vi "Arm_Control.vi"() -> ()   [LabVIEW 2012]
uses:
  StateMachineType.ctl
  Robot Global Data.vi
panel:
  in  "ArmBackSpeed":dbl=-0.32
  in  "ArmForwardSpeed":dbl=0.32
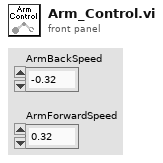
[diagram p1: front panel]
types:
  T1 = typedef "StateMachineType.ctl" = enum16{"Init", "Idle", "Start", "Do", "Stop"}
  T2 = typedef "WPI_MotorControlDeviceRef.ctl" = cluster{"DeviceStatus":errorcluster, "Type":enum16{"PWM", "CAN"}, "PWM":cluster{"Digital Module":T3, "PWM Channel":T4, "DeadBand":T5}, "CAN":cluster{"Device Number":u8, "Control Mode":T6, "Semaphore":T7, "Max Vout":dbl}, "Invert":bool, "TransformRef":T8, "InvTransformRef":T8}
  T3 = typedef "FPGA_TypedefDigitalModule.ctl" = enum16{"Digital Module 1", "Digital Module 2"}
  T4 = typedef "FPGA_DIOPWMChannel.ctl" = enum8{"PWM 1", "PWM 2", "PWM 3", "PWM 4", "PWM 5", "PWM 6", "PWM 7", "PWM 8", "PWM 9", "PWM 10", "Invalid"}
  T5 = typedef "WPI_PWMDeadband.ctl" = cluster{"Name":string, "maxPositivePwm":i32, "minPositivePwm":i32, "centerPwm":i32, "maxNegativePwm":i32, "minNegativePwm":i32, "angularRange":u16}
  T6 = typedef "WPI_CANJaguar_ControlMode.ctl" = enum8{"Percent VBus", "Current", "Speed", "Position", "Voltage"}
  T7 = typedef "Semaphore RefNum" = refnum<k1>
  T8 = typedef "WPI_PWMTransform_ConPane.ctl" = refnum<vi>
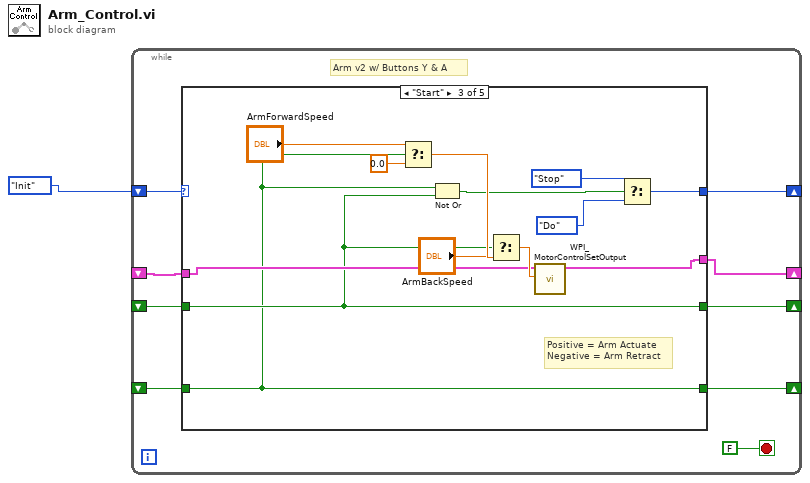
[diagram p0: block diagram]
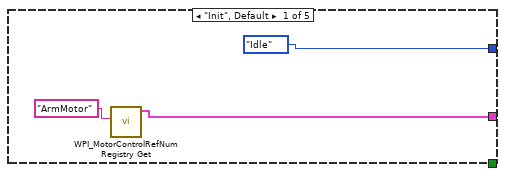
[diagram p2: hidden frame]
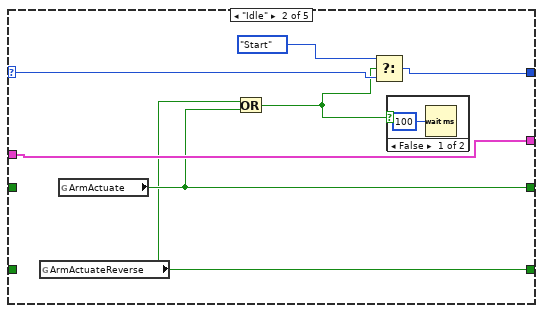
[diagram p3: hidden frame]
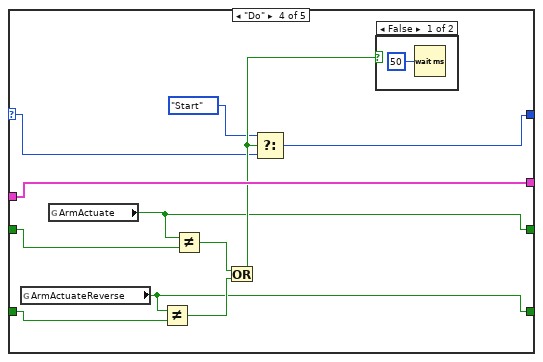
[diagram p5: hidden frame]
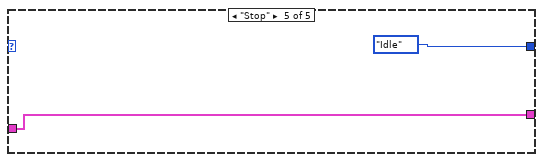
[diagram p7: hidden frame]
diagram:
  n1 = while {
    shift-right: [w6] -> _
    shift-left: _ -> [w9]
    shift-right: [w7] -> _
    shift-left: StateMachineType."Init" -> [w8]
    shift-right: [w4] -> _
    shift-left: _ -> [w2]
    shift-right: [w5] -> _
    shift-left: _ -> [w3]
    stop <- FALSE stop-if-true
    # "Arm v2 w/ Buttons Y & A"
    n2 = case shown="\"Start\"" w8 {
      selector: w8 -> [_ w20 _ w35 _]
      tunnel: w9 -> [_ w17 w24 w45 w47]
      tunnel: [StateMachineType."Idle" ("Enum") w18 w26 w39 StateMachineType."Idle" ("Enum")] -> w7
      tunnel: [w11 w17 w25 w45 w47] -> w6
      tunnel: [_ w15 w23 w38 _] -> w5
      tunnel: [_ w14 w22 w37 _] -> w4
      tunnel: w3 -> [_ _ w23 w44 _]
      tunnel: w2 -> [_ _ w22 w43 _]
      frame "Init", Default {
        n3 = call <vilib>:"WPI_MotorControlRefNum Registry Get.vi"("refnum name"="ArmMotor") -> ("MotorControlDevRef"=w11:T2)  [unwired: 9 in, 1 out]
      }
      frame "Idle" {
        n4 = global read "Robot Global Data.vi" "ArmActuateReverse"() -> (w14:bool)
        n5 = global read "Robot Global Data.vi" "ArmActuate"() -> (w15:bool)
        n6 = Or(x=w14, y=w15) -> (x .or. y?=w16:bool)
        n7 = Select(t=StateMachineType."Start" ("Enum"), s=w16, f=w20) -> (s? t:f=w18:T1)
        n8 = case shown="False" w16 {
          frame False {
            n9 = Wait (ms)(milliseconds to wait=u32 100) -> ()  [unwired: 1 out]
          }
          frame True {
          }
        }
      }
      frame "Start" {
        # "Positive = Arm Actuate\nNegative = Arm Retract"
        n10 = Select(t="ArmForwardSpeed", s=w22, f=0.0) -> (s? t:f=w34:dbl)
        n11 = Not Or(1:w23, 2:w22) -> (0:w31:bool)
        n12 = Select(t="ArmBackSpeed", s=w23, f=w34) -> (s? t:f=w30:dbl)
        n13 = call <vilib>:"WPI_MotorControlSetOutput.vi"("Output"=w30, "MotorControlDevRef"=w24) -> ("MotorControlDevRef"=w25:T2)  [unwired: 7 in, 2 out]
        n14 = Select(t=StateMachineType."Stop" ("Enum"), s=w31, f=StateMachineType."Do" ("Enum")) -> (s? t:f=w26:T1)
      }
      frame "Do" {
        n15 = global read "Robot Global Data.vi" "ArmActuateReverse"() -> (w37:bool)
        n16 = global read "Robot Global Data.vi" "ArmActuate"() -> (w38:bool)
        n17 = Not Equal?(x=w37, y=w43) -> (x != y?=w41:bool)
        n18 = Not Equal?(x=w38, y=w44) -> (x != y?=w42:bool)
        n19 = Or(x=w42, y=w41) -> (x .or. y?=w40:bool)
        n20 = Select(t=StateMachineType."Start" ("Enum"), s=w40, f=w35) -> (s? t:f=w39:T1)
        n21 = case shown="False" w40 {
          frame False {
            n22 = Wait (ms)(milliseconds to wait=u32 50) -> ()  [unwired: 1 out]
          }
          frame True {
          }
        }
      }
      frame "Stop" {
      }
    }
  }
